vi "Global communication output.vi"() -> ()   [LabVIEW 2016]
panel:
  in  "PV Control":dbl[](array[numeric])
  in  "BESS Control":dbl[](array[numeric])
  in  "IntellRupter Control":bool[](array[boolean])
  in  "Matrix output":bool
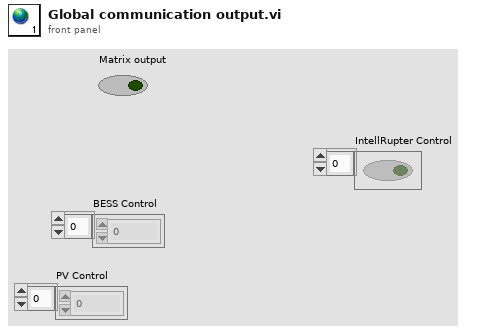
[diagram p1: front panel]
diagram:
